vi "Logon GUI.vi"(4 "updated user":bool, 6 "valid form":bool, 8 "logon status":T3=enum."unregistered email", 9 "User Information from db":T1 {"Country" items=["Afghanistan", "Aland Islands", "Albania", "Algeria", "American Samoa", "Andorra", "Angola", "Anguilla", "Antarctica", "Antigua And Barbuda", "Argentina", "Armenia", "Aruba", "Australia", "Austria", "Azerbaijan", "Bahamas", "Bahrain", "Bangladesh", "Barbados", "Belarus", "Belgium", "Belize", "Benin", "Bermuda", "Bhutan", "Bolivia", "Bosnia And Herzegovina", "Botswana", "Bouvet Island", "Brazil", "British Indian Ocean Territory", "Brunei Darussalam", "Bulgaria", "Burkina Faso", "Burundi", "Cambodia", "Cameroon", "Canada", "Cape Verde", "Cayman Islands", "Central African Republic", "Chad", "Chile", "China", "Christmas Island", "Cocos (Keeling) Islands", "Colombia", "Comoros", "Congo", "Congo, The Democratic Republic Of The", "Cook Islands", "Costa Rica", "Cote D'Ivoire", "Croatia", "Cuba", "Cyprus", "Czech Republic", "Denmark", "Djibouti", "Dominica", "Dominican Republic", "Ecuador", "Egypt", "El Salvador", "Equatorial Guinea", "Eritrea", "Estonia", "Ethiopia", "Falkland Islands (Malvinas)", "Faroe Islands", "Fiji", "Finland", "France", "French Guiana", "French Polynesia", "French Southern Territories", "Gabon", "Gambia", "Georgia", "Germany", "Ghana", "Gibraltar", "Greece", "Greenland", "Grenada", "Guadeloupe", "Guam", "Guatemala", "Guernsey", "Guinea", "Guinea-Bissau", "Guyana", "Haiti", "Heard Island And Mcdonald Islands", "Holy See (Vatican City State)", "Honduras", "Hong Kong", "Hungary", "Iceland", "India", "Indonesia", "Iran, Islamic Republic Of", "Iraq", "Ireland", "Isle Of Man", "Israel", "Italy", "Jamaica", "Japan", "Jersey", "Jordan", "Kazakhstan", "Kenya", "Kiribati", "Korea, Democratic People'S Republic Of", "Korea, Republic Of", "Kuwait", "Kyrgyzstan", "Lao People'S Democratic Republic", "Latvia", "Lebanon", "Lesotho", "Liberia", "Libyan Arab Jamahiriya", "Liechtenstein", "Lithuania", "Luxembourg", "Macao", "Macedonia, The Former Yugoslav Republic Of", "Madagascar", "Malawi", "Malaysia", "Maldives", "Mali", "Malta", "Marshall Islands", "Martinique", "Mauritania", "Mauritius", "Mayotte", "Mexico", "Micronesia, Federated States Of", "Moldova, Republic Of", "Monaco", "Mongolia", "Montserrat", "Morocco", "Mozambique", "Myanmar", "Namibia", "Nauru", "Nepal", "Netherlands", "Netherlands Antilles", "New Caledonia", "New Zealand", "Nicaragua", "Niger", "Nigeria", "Niue", "Norfolk Island", "Northern Mariana Islands", "Norway", "Oman", "Pakistan", "Palau", "Palestinian Territory, Occupied", "Panama", "Papua New Guinea", "Paraguay", "Peru", "Philippines", "Pitcairn", "Poland", "Portugal", "Puerto Rico", "Qatar", "Reunion", "Romania", "Russian Federation", "Rwanda", "Saint Helena", "Saint Kitts And Nevis", "Saint Lucia", "Saint Pierre And Miquelon", "Saint Vincent And The Grenadines", "Samoa", "San Marino", "Sao Tome And Principe", "Saudi Arabia", "Senegal", "Serbia And Montenegro", "Seychelles", "Sierra Leone", "Singapore", "Slovakia", "Slovenia", "Solomon Islands", "Somalia", "South Africa", "South Georgia And The South Sandwich Islands", "Spain", "Sri Lanka", "Sudan", "Suriname", "Svalbard And Jan Mayen", "Swaziland", "Sweden", "Switzerland", "Syrian Arab Republic", "Taiwan, Province Of China", "Tajikistan", "Tanzania, United Republic Of", "Thailand", "Timor-Leste", "Togo", "Tokelau", "Tonga", "Trinidad And Tobago", "Tunisia", "Turkey", "Turkmenistan", "Turks And Caicos Islands", "Tuvalu", "Uganda", "Ukraine", "United Arab Emirates", "United Kingdom", "United States", "United States Minor Outlying Islands", "Uruguay", "Uzbekistan", "Vanuatu", "Venezuela", "Viet Nam", "Virgin Islands, British", "Virgin Islands, U.S.", "Wallis And Futuna", "Western Sahara", "Yemen", "Zambia", "Zimbabwe", "(Not Specified)"]}, 10 "User Options":refnum<vi>, 11 "User Info":refnum<vi>) -> ()   [LabVIEW 2015, in "AguaClara Library.lvlib"]
uses:
  AguaClara Library.lvlib
  User status.ctl
  User Information.ctl
  Country Ring.ctl
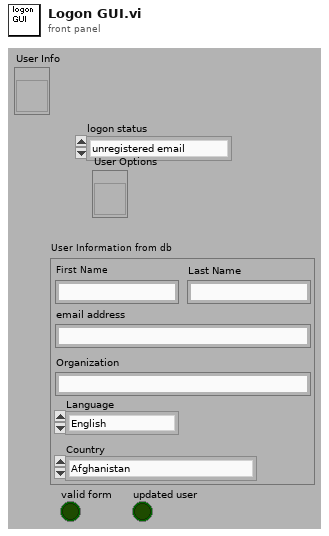
[diagram p1: front panel]
types:
  T1 = typedef "AguaClara Library.lvlib/User Information.ctl" = cluster{"First Name":string, "Last Name":string, "Email Address":string, "Organization":string, "Language":enum16{"English", "Español", "French"}, "Country":T2}
  T2 = typedef "Country Ring.ctl" = u16
  T3 = typedef "AguaClara Library.lvlib/User status.ctl" = enum16{"invalid email", "unregistered email", "registered email"}
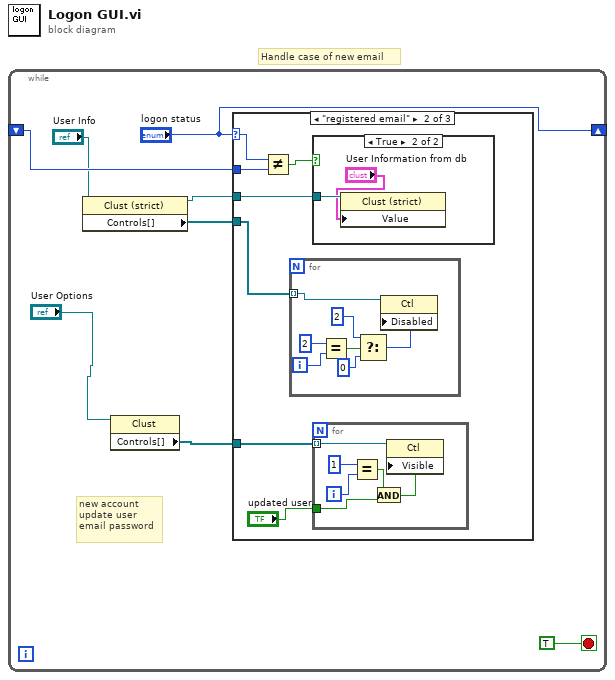
[diagram p0: block diagram]
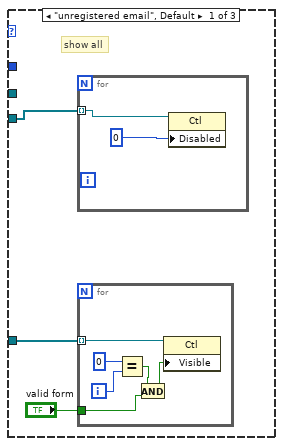
[diagram p2: hidden frame]
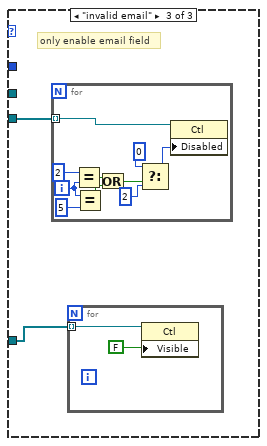
[diagram p4: hidden frame]
diagram:
  # "Handle case of new email"
  n1 = while {
    shift-right: ["logon status"] -> _
    shift-left: _ -> [w7]
    stop <- TRUE stop-if-true
    # "new account\nupdate user\nemail password"
    n2 = property class="Clust (strict)"(reference="User Info") -> (reference out=w5:refnum<vi>, "Controls[]"=w8:refnum<vi>[])  [unwired: 1 in, 1 out]
    n3 = property class="Clust"(reference="User Options") -> ("Controls[]"=w3:refnum<vi>[])  [unwired: 1 in, 2 out]
    n4 = case shown="\"registered email\"" "logon status" {
      selector: "logon status" -> [_ w24 _]
      tunnel: w8 -> [w11 w26 w43]
      tunnel: w7 -> [_ w25 _]
      tunnel: w5 -> [_ w22 _]
      tunnel: w3 -> [w10 w21 w42]
      frame "unregistered email", Default {
        # "show all"
        n5 = for {
          tunnel: w11 -> [w19] mode=indexing
          n6 = property class="Ctl"(reference=w19, "Disabled"=u8 0) -> ()  [unwired: 1 in, 2 out]
        }
        n7 = for {
          tunnel: w10 -> [w17] mode=indexing
          tunnel: "valid form" -> [w13]
          i -> [w16]
          n8 = Equal?(x=0, y=w16) -> (x = y?=w14:bool)
          n9 = And(x=w14, y=w13) -> (x .and. y?=w12:bool)
          n10 = property class="Ctl"(reference=w17, "Visible"=w12) -> ()  [unwired: 1 in, 2 out]
        }
      }
      frame "registered email" {
        n11 = Not Equal?(x=w24, y=w25) -> (x != y?=w23:bool)
        n12 = for {
          tunnel: w26 -> [w41] mode=indexing
          i -> [w36]
          n13 = Equal?(x=2, y=w36) -> (x = y?=w39:bool)
          n14 = Select(t=u8 2 ("Disabled"), s=w39, f=u8 0 ("Disabled")) -> (s? t:f=w35:u8)
          n15 = property class="Ctl"(reference=w41, "Disabled"=w35) -> ()  [unwired: 1 in, 2 out]
        }
        n16 = case shown="True" w23 {
          tunnel: w22 -> [_ w34]
          frame False {
          }
          frame True {
            n17 = property class="Clust (strict)"(reference=w34, "Value"="User Information from db") -> ()  [unwired: 1 in, 2 out]
          }
        }
        n18 = for {
          tunnel: w21 -> [w32] mode=indexing
          tunnel: "updated user" -> [w28]
          i -> [w31]
          n19 = Equal?(x=1, y=w31) -> (x = y?=w29:bool)
          n20 = And(x=w29, y=w28) -> (x .and. y?=w27:bool)
          n21 = property class="Ctl"(reference=w32, "Visible"=w27) -> ()  [unwired: 1 in, 2 out]
        }
      }
      frame "invalid email" {
        # "only enable email field"
        n22 = for {
          tunnel: w43 -> [w53] mode=indexing
          i -> [w48]
          n23 = Equal?(x=2, y=w48) -> (x = y?=w54:bool)
          n24 = Equal?(x=w48, y=5 ("x")) -> (x = y?=w47:bool)
          n25 = Or(x=w54, y=w47) -> (x .or. y?=w49:bool)
          n26 = Select(t=u8 0 ("Disabled"), s=w49, f=u8 2 ("Disabled")) -> (s? t:f=w52:u8)
          n27 = property class="Ctl"(reference=w53, "Disabled"=w52) -> ()  [unwired: 1 in, 2 out]
        }
        n28 = for {
          tunnel: w42 -> [w45] mode=indexing
          n29 = property class="Ctl"(reference=w45, "Visible"=FALSE) -> ()  [unwired: 1 in, 2 out]
        }
      }
    }
  }
